vi "Is_Idle.vi"(8 "error in (no error)":errorcluster, 11 "Up/Down/Idle":T1) -> (0 "error out":errorcluster, 3 "score":i32)   [LabVIEW 2026]
uses:
  Controls/Motion_Status_Enum.ctl
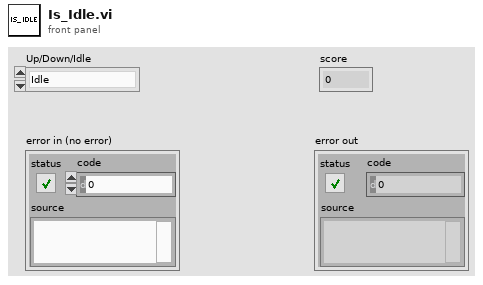
[diagram p1: front panel]
types:
  T1 = typedef "Motion_Status_Enum.ctl" = enum16{"Idle", "Up", "Down"}
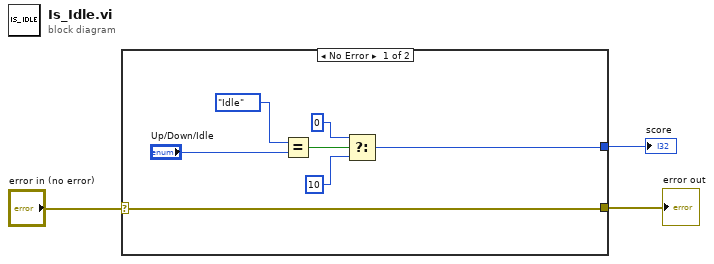
[diagram p0: block diagram]
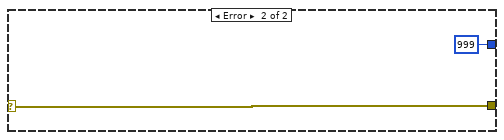
[diagram p2: hidden frame]
diagram:
  n1 = case shown="No Error" "error in (no error)" {
    selector: "error in (no error)" -> [w4 w12]
    tunnel: [w5 999 ("y")] -> w2
    tunnel: [w4 w12] -> w1
    frame No Error {
      n2 = Equal?(x=Motion_Status_Enum."Idle" ("Up/Down"), y="Up/Down/Idle") -> (x = y?=w8:bool)
      n3 = Select(t=0 ("y"), s=w8, f=10 ("y")) -> (s? t:f=w5:i32)
    }
    frame Error {
    }
  }
  "error out" <- w1
  "score" <- w2
